vi "AnkleLocHistory.vi"(1 "history length (100)":i32=100, 2 "AnkleLoc":dbl[](array[numeric]), 4 "initialize":bool) -> (5 "AnkleLoc":dbl[][](array[numeric]))   [LabVIEW 2015]
uses:
  <vilib>/ptbypt/NI_PtbyPt.lvlib
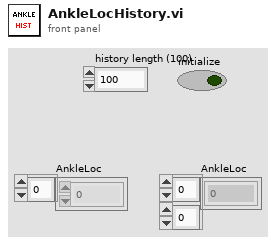
[diagram p1: front panel]
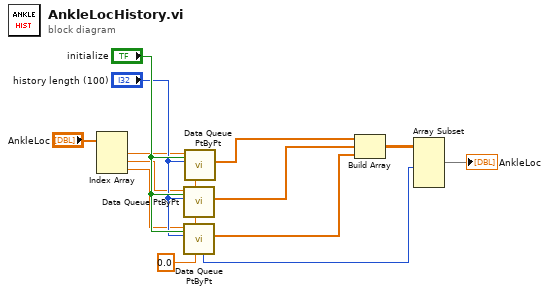
[diagram p0: block diagram]
diagram:
  w10 = 0.0 ("initial queue element")
  n1 = Index Array(array="AnkleLoc") -> (element #1=w4:dbl, element #2=w5:dbl, element #3=w7:dbl)  [unwired: 3 in]
  n2 = call <vilib>:"Data Queue PtByPt.vi"("initial queue element"=w10, "initialize"="initialize", "sample length"="history length (100)", "input data point"=w5) -> ("Current Queue"=w12:dbl[])  [unwired: 3 in, 4 out]
  n3 = call <vilib>:"Data Queue PtByPt.vi"("initial queue element"=w10, "initialize"="initialize", "sample length"="history length (100)", "input data point"=w7) -> ("Current Queue"=w13:dbl[], "current length"=w2:i32)  [unwired: 3 in, 3 out]
  n4 = call <vilib>:"Data Queue PtByPt.vi"("initial queue element"=w10, "initialize"="initialize", "sample length"="history length (100)", "input data point"=w4) -> ("Current Queue"=w11:dbl[])  [unwired: 3 in, 4 out]
  n5 = Build Array(w11, w12, w13) -> (w3:dbl[][])
  n6 = Array Subset(array=w3, length (row)=w2) -> (→"AnkleLoc":dbl[][])  [unwired: 3 in]
